vi "KM_ControlHFLI.vi"(4 "Control HFLI command":T2=enum."Scan frequency", 8 "ZI HFLI System Parameters IN":T1={"IP Address"="DEV987", "Start (Hz)"=10000.0, "Stop (Hz)"=1000000.0, "Filter Order"=4, "Number of Points"=100, "Precision"=0, "Bandwidth (Hz)"=-1.0, "Averaging"=1, "Log Sweep"=FALSE, "Demod"=3} {"Averaging" items=["1"=1, "2"=2, "4"=4, "16"=16, "32"=32, "64"=64]; "Bandwidth (Hz)" format="%#_p"; "Precision" items=["Low", "Med", "High"]; "Number of Points" min=2 max=66000; "Filter Order" items=["6, 1st"=1, "12, 2nd"=2, "18, 3rd"=3, "24, 4th"=4, "30, 5th"=5, "36, 6th"=6, "42, 7th"=7, "48, 8th"=8]; "Stop (Hz)" format="%_5p"; "Start (Hz)" format="%_5p"}) -> (0 "Voltage out":cdb[](array[numeric]), 1 "Freq out":dbl[](array[numeric]), 3 "ZI HFLI System Parameters OUT":T1={"IP Address"="DEV987", "Start (Hz)"=10000.0, "Stop (Hz)"=1000000.0, "Filter Order"=4, "Number of Points"=100, "Precision"=0, "Bandwidth (Hz)"=-1.0, "Averaging"=1, "Log Sweep"=FALSE, "Demod"=3} {"Averaging" items=["1"=1, "2"=2, "4"=4, "16"=16, "32"=32, "64"=64]; "Bandwidth (Hz)" format="%#_p"; "Precision" items=["Low", "Med", "High"]; "Number of Points" min=2 max=66000; "Filter Order" items=["6, 1st"=1, "12, 2nd"=2, "18, 3rd"=3, "24, 4th"=4, "30, 5th"=5, "36, 6th"=6, "42, 7th"=7, "48, 8th"=8]; "Stop (Hz)" format="%_5p"; "Start (Hz)" format="%_5p"})   [LabVIEW 2016]
doc: "Control a Zurich instrument device via the LabOne Labview API. \nRequirements: Zurich Instruments HF2 (HF2IS or HF2LI-MF ).\nThis example uses the API functions to perform a frequency sweep and measure the impedance. \n\n© Zurich Instruments AG, www.zhinst.com"
uses:
  KM_ControlHFLIcommand.ctl
  KM_SystemParameters.ctl
  Zurich/Zurich Instruments/LabOne/API/LabVIEW/Zurich Instruments LabOne/Zurich Instruments LabOne.lvlib
panel:
  out "Current out":cdb[](array[numeric])
  out "Point 2":i32=10 caption="Point (#)"
  out "cal_types":cluster{string[], bool[]}[](array[cluster])=[{["R (Ohms)", " ", " "], [TRUE, FALSE, FALSE]}, {["C (F)", " ", " "], [TRUE, FALSE, FALSE]}, {["L (H)", " ", " "], [TRUE, FALSE, FALSE]}, {["R (Ohms)", "C (F)\n ", " "], [TRUE, TRUE, FALSE]}]
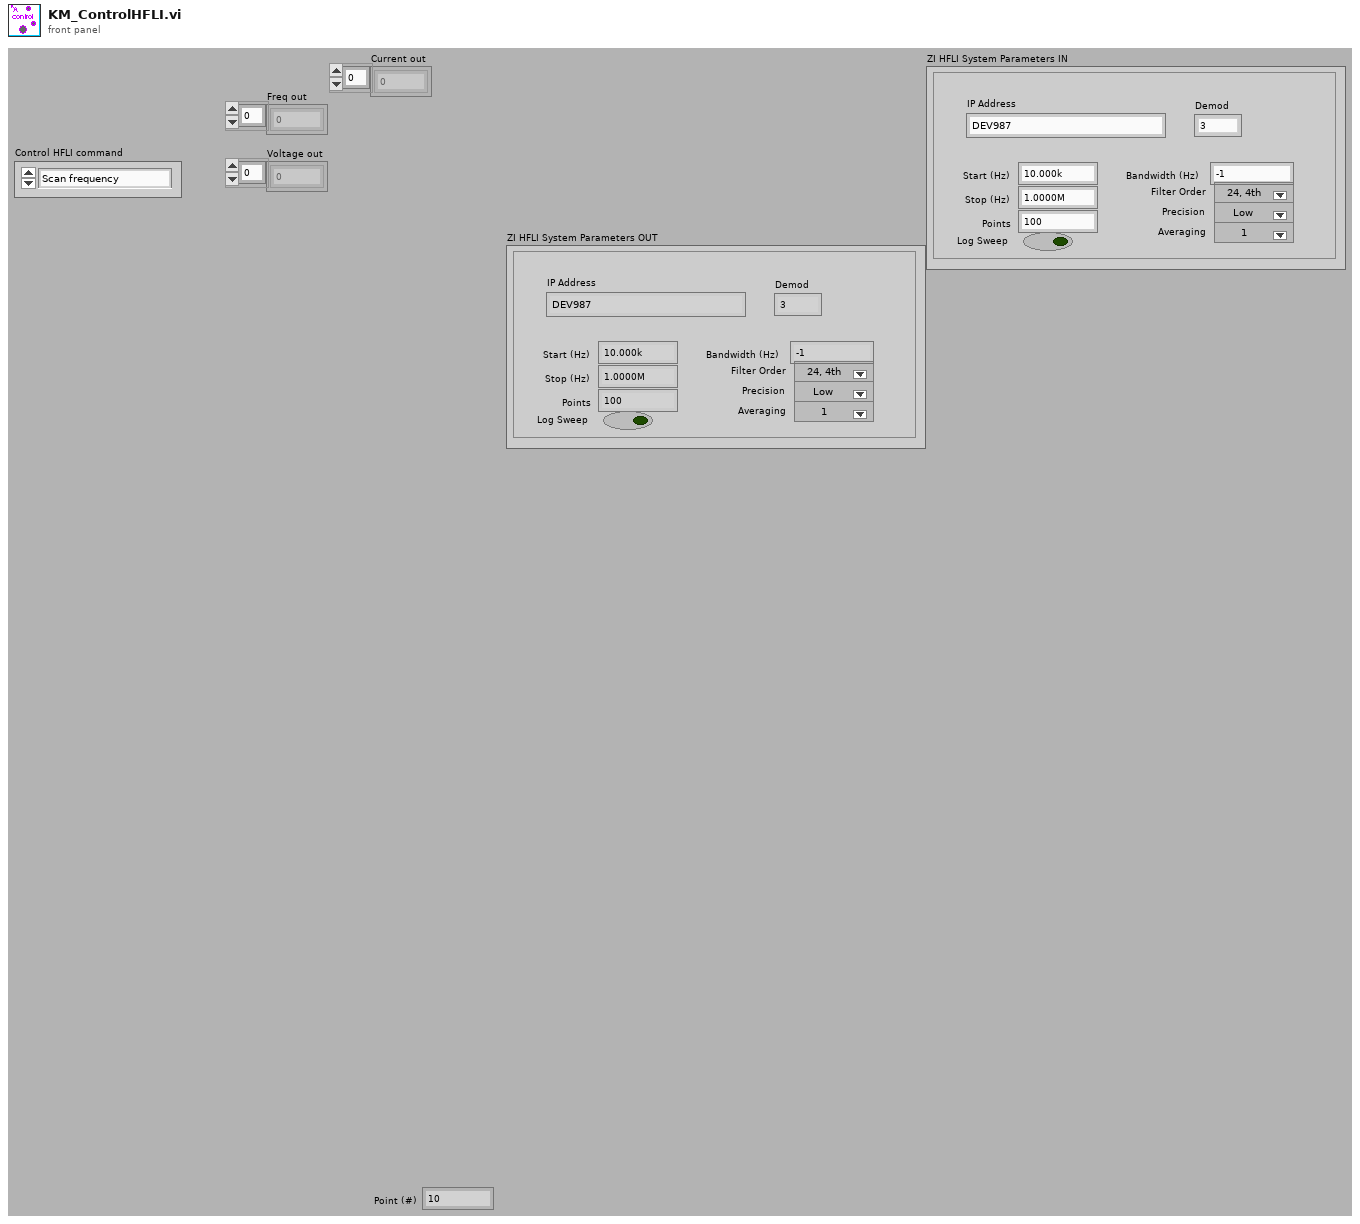
[diagram p1: front panel]
types:
  T1 = typedef "KM_SystemParameters.ctl" = cluster{"IP Address":string, "Start (Hz)":dbl, "Stop (Hz)":dbl, "Filter Order":i32, "Number of Points":i32, "Precision":u16, "Bandwidth (Hz)":dbl, "Averaging":u16, "Log Sweep":bool, "Demod":i32}
  T2 = typedef "KM_ControlHFLIcommand.ctl" = enum16{"Initialize", "Scan frequency"}
  T3 = cluster{"Output (F,X1,Y1,X2,Y2,...,Vo)":dbl[][], "Point (#)":i32}
  T4 = typedef "Zurich Instruments LabOne.lvlib/ziTypeHandle.ctl" = cluster{"handleValid":bool, "Conn":u64, "Path Prefix":string, "Handle":u64, "Connected":bool, "Clockbase(s)":dbl}
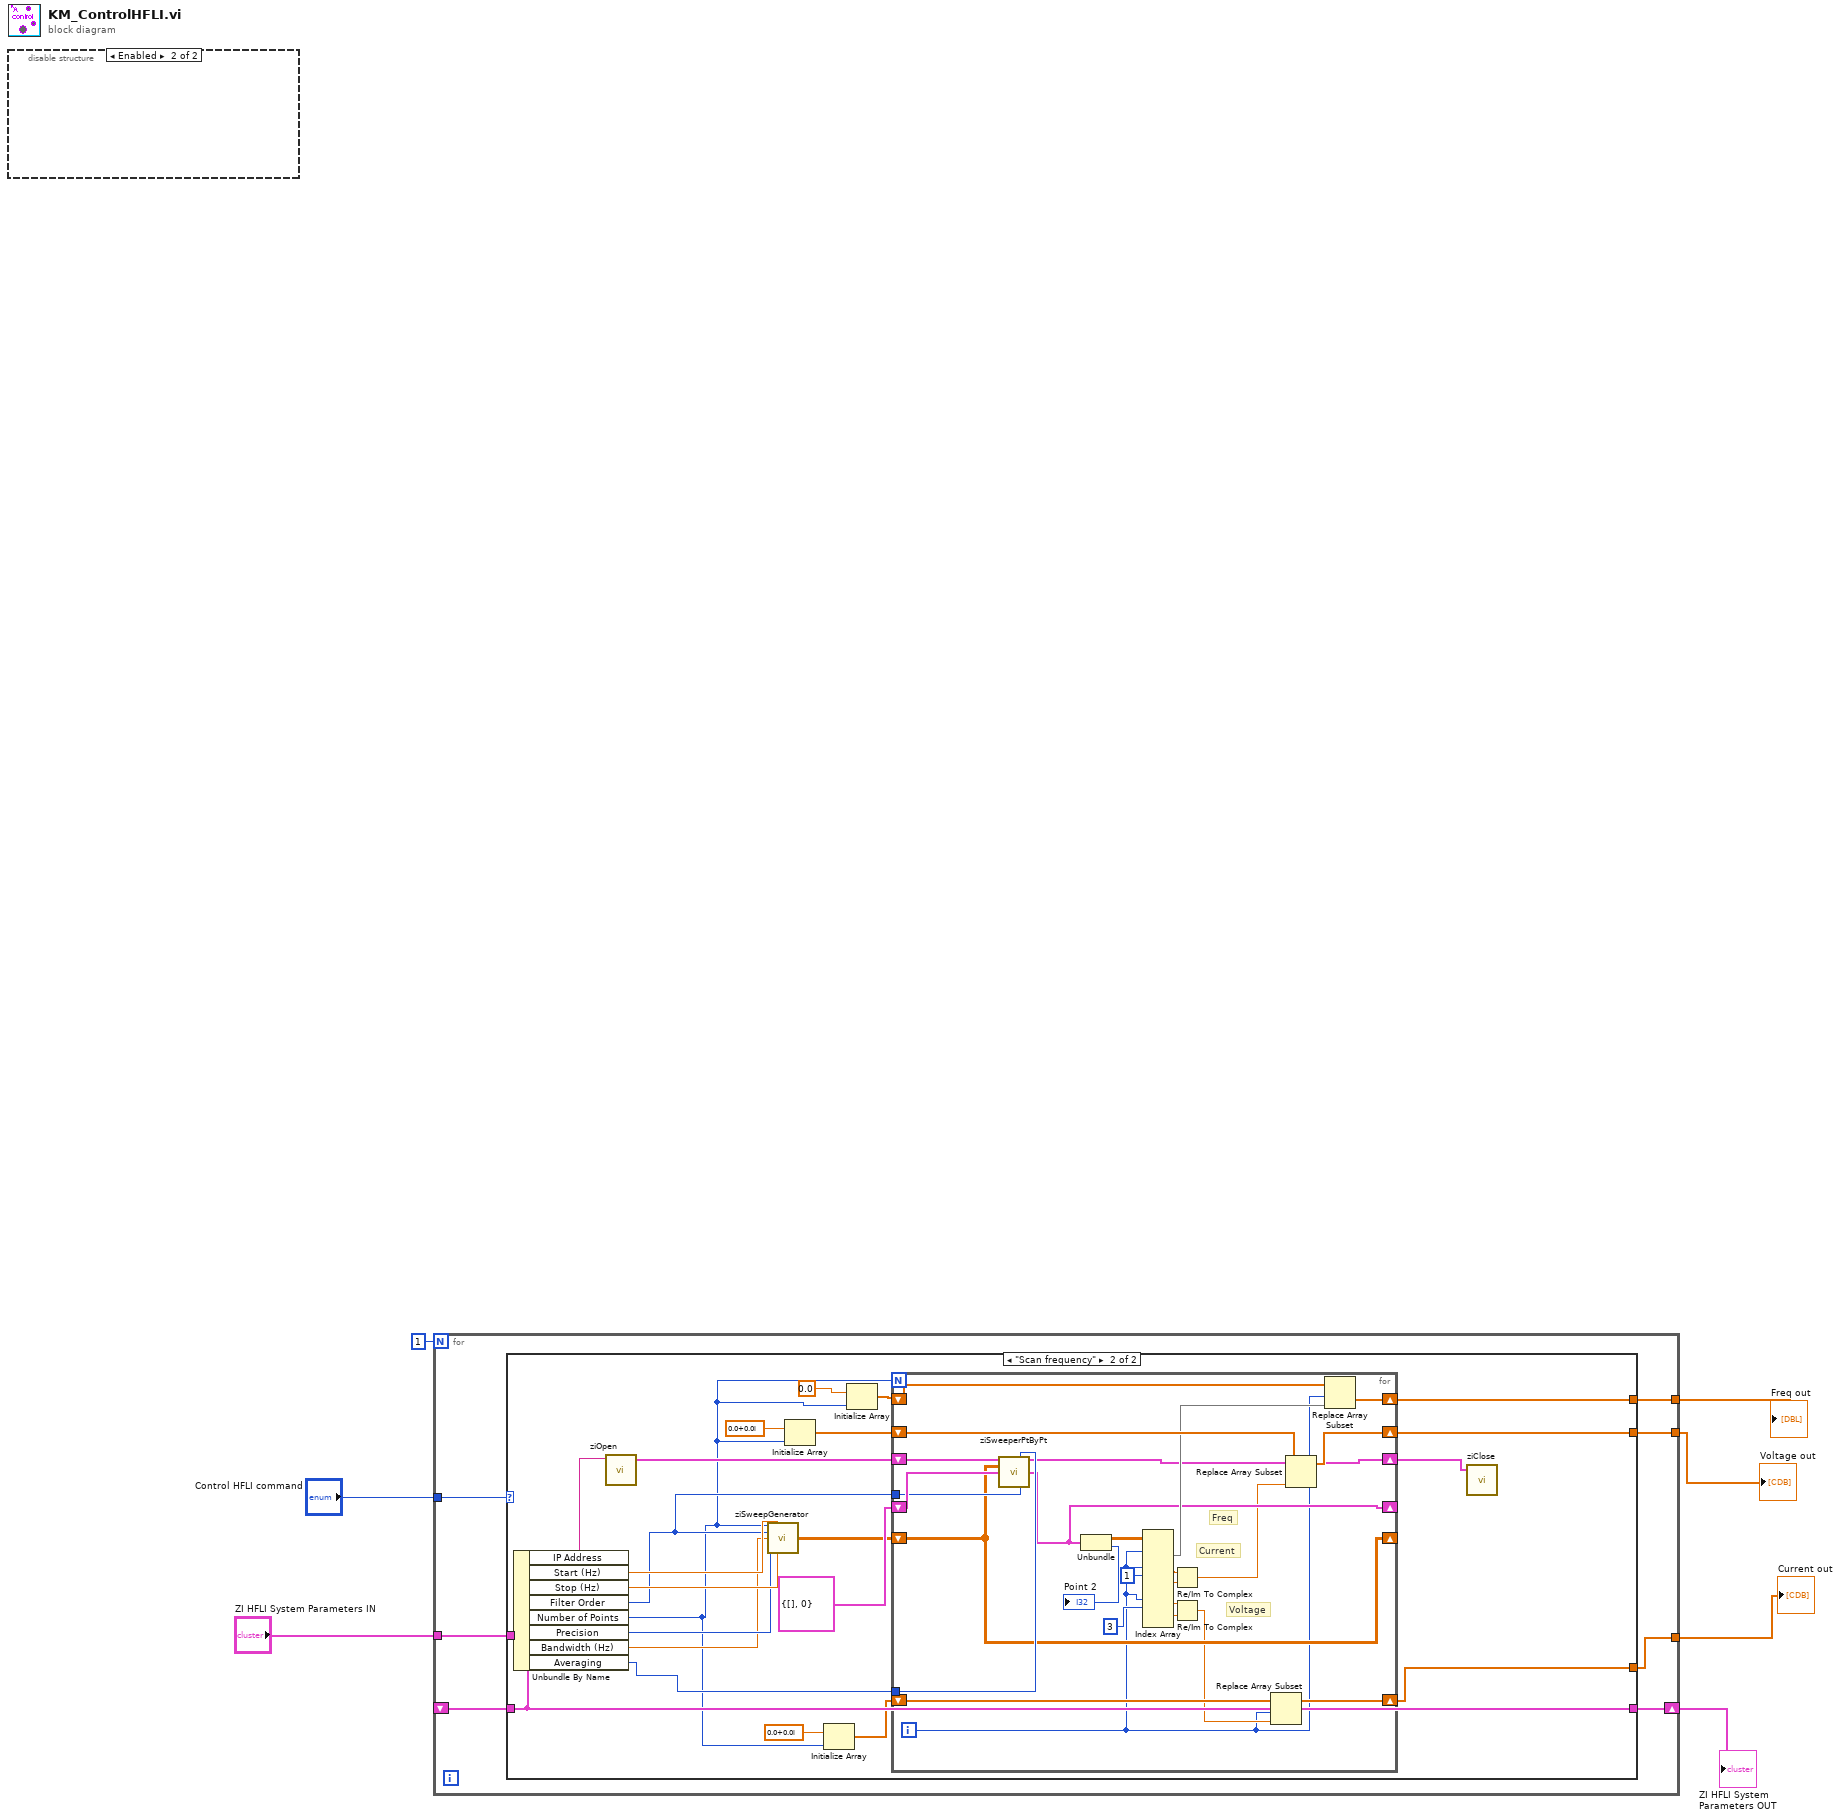
[diagram p0: block diagram]
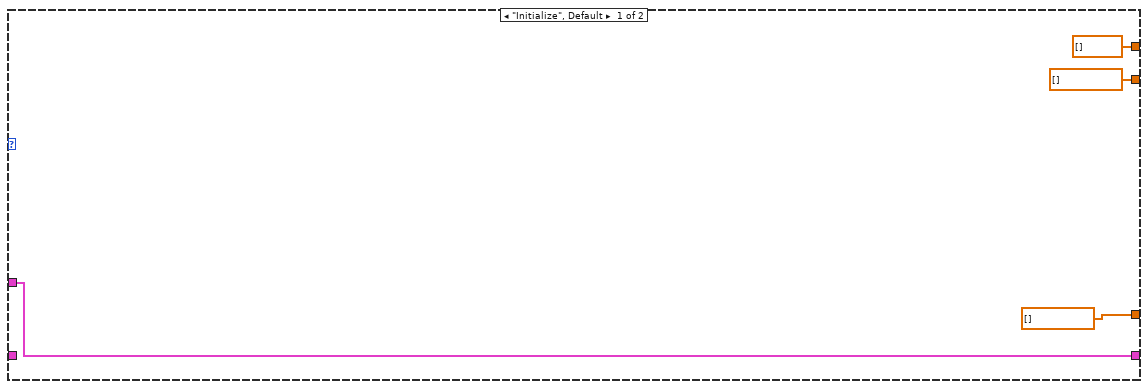
[diagram p2: hidden frame]
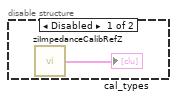
[diagram p3: hidden frame]
diagram:
  n1 = disable-structure shown="Enabled" {
    frame Disabled {
      n2 = call <instrlib>:"ziImpedanceCalibRefZ.vi"() -> ("cal_types"=→"cal_types":cluster{string[], bool[]}[], 2:w8)  [unwired: 3 in, 1 out]
    }
    frame Enabled {
    }
  }
  n3 = for {
    N: 1 -> [_]
    tunnel: "Control HFLI command" -> [w16]
    tunnel: "ZI HFLI System Parameters IN" -> [w15]
    shift-right: [w14] -> w3
    shift-left: _ -> [w13]
    tunnel: [w12] -> w5
    tunnel: [w11] -> w4
    tunnel: [w10] -> w2
    n4 = case shown="\"Scan frequency\"" w16 {
      tunnel: w15 -> [w20 _]
      tunnel: [w20 w42] -> w14
      tunnel: w13 -> [_ w42]
      tunnel: [dbl[] [] w26] -> w12
      tunnel: [cdb[] [] w25] -> w11
      tunnel: [cdb[] [] w21] -> w10
      frame "Initialize", Default {
      }
      frame "Scan frequency" {
        n5 = Unbundle By Name(w42) -> ("IP Address"=w41:string, "Start (Hz)"=w40:dbl, "Stop (Hz)"=w39:dbl, "Filter Order"=w32:i32, "Number of Points"=w22:i32, "Precision"=w38:u16, "Bandwidth (Hz)"=w37:dbl, "Averaging"=w31:u16)
        n6 = call "ziOpen.vi"("Address"=w41) -> ("HandleOut"=w28:T4)  [unwired: 3 in, 2 out]
        n7 = call "ziSweepGenerator.vi"("Steps (#)"=w22, "Start (Hz)"=w40, "Order (4)"=w32, "Bandwith (-1=auto)"=w37, "Precision (Low)"=w38, "Stop (Hz)"=w39) -> ("Sweep Sequence (F (Hz), BW (Hz), TC(s), Time(s))"=w33:dbl[][])  [unwired: 7 in, 2 out]
        n8 = Initialize Array(cdb 0.0+0.0i ("element"), w22) -> (w35:cdb[])
        n9 = Initialize Array(cdb 0.0+0.0i ("element"), w22) -> (w23:cdb[])
        n10 = Initialize Array(0.0 ("element"), w22) -> (w29:dbl[])
        n11 = for {
          N: w22 -> [_]
          shift-right: [w66] -> w25
          shift-left: w35 -> [w67]
          shift-right: [w50] -> _
          shift-left: T3 {"Output (F,X1,Y1,X2,Y2,...,Vo)"=[], "Point (#)"=0} ("State Out") -> [w65]
          shift-right: [w51] -> _
          shift-left: w33 -> [w51]
          tunnel: w32 -> [w64]
          tunnel: w31 -> [w63]
          shift-right: [w55] -> w26
          shift-left: w29 -> [w56]
          shift-right: [w53] -> w27
          shift-left: w28 -> [w52]
          shift-right: [w45] -> w21
          shift-left: w23 -> [w46]
          i -> [w43]
          # "Voltage"
          # "Current"
          # "Freq"
          n12 = call "ziSweeperPtByPt.vi"("Handle In"=w52, "Averaging"=w63, "Sweep Sequence In"=w51, "State In"=w65, "Order (4)"=w64) -> ("Handle Out"=w53:T4, "State Out"=w50:T3)  [unwired: 7 in, 2 out]
          n13 = Unbundle(w50) -> ("Output (F,X1,Y1,X2,Y2,...,Vo)"=w57:dbl[][], "Point (#)"=→"Point 2":i32)
          n14 = Index Array(array=w57, index (row) #1=w43, index (row) #2=w43, index (col) #2=1 ("disabled index (col)"), index (row) #4=w43, index (col) #4=3 ("disabled index (col)")) -> (element #1=w54:dbl[], element #2=w61:dbl, element #3=w62:dbl, element #4=w60:dbl, element #5=w59:dbl)  [unwired: 5 in]
          n15 = Re/Im To Complex(1:w62, 2:w61) -> (0:w49:cdb)
          n16 = Re/Im To Complex(1:w59, 2:w60) -> (0:w44:cdb)
          n17 = Replace Array Subset(array=w46, new element=w44, index=w43) -> (w45:cdb[])
          n18 = Replace Array Subset(array=w67, new element=w49, index=w43) -> (w66:cdb[])
          n19 = Replace Array Subset(array=w56, new element=w54, index=w43) -> (w55:dbl[])
        }
        n20 = call "ziClose.vi"("Handle In"=w27) -> ()  [unwired: 3 in, 2 out]
      }
    }
  }
  "Freq out" <- w5
  "Voltage out" <- w4
  "ZI HFLI System Parameters OUT" <- w3
  "Current out" <- w2
